vi "Check Error Core.vi"(8 "error in (no error)":errorcluster, 11 "Error Code":i32) -> (0 "error out":errorcluster)   [LabVIEW 2021, in "CIF_NI_CIPC.lvlib"]
doc: "This core VI is only called if an error exists. This is set for more effecient memory usage to not be reentrant."
uses:
  CIF_NI_CIPC.lvlib
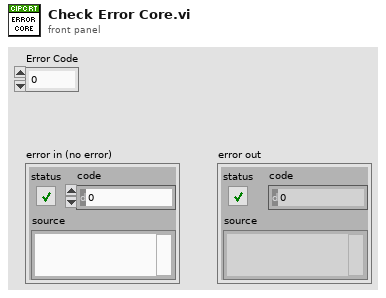
[diagram p1: front panel]
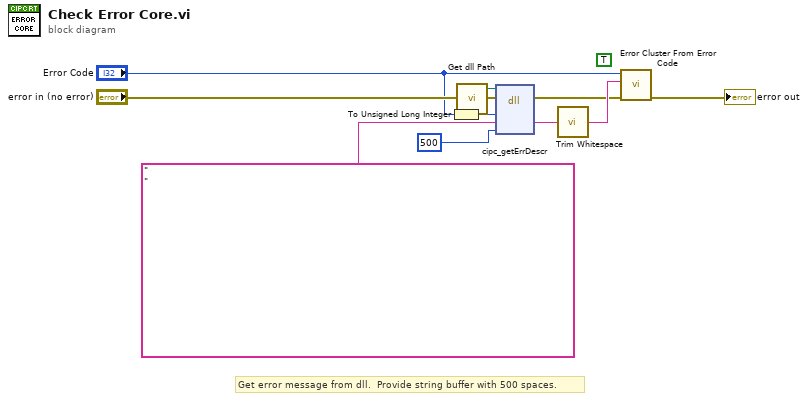
[diagram p0: block diagram]
diagram:
  (unwired) TRUE ("show call chain? (False)")
  # "Get error message from dll.  Provide string buffer with 500 spaces."
  n1 = To Unsigned Long Integer(number="Error Code") -> (unsigned 32bit integer=w8:u32)
  n2 = call "Get dll Path.vi"() -> ("appended path"=w10:path)  [unwired: 5 in]
  n3 = dll-call lib="libnicipc.*" fn="cipc_getErrDescr"(path in=w10, error in="error in (no error)", "err_code"=w8, "el_descr"="                                                                                                                                                                                                                                                                                                                                                                                                                                                                                                                    " ("string"), "el_descr_maxsize"=u32 500 ("dimension size")) -> (error out=w6:errorcluster, "el_descr"=w5:string)  [unwired: 4 in, 1 out]
  n4 = call <vilib>:"Trim Whitespace.vi"("string"=w5) -> ("trimmed string"=w9:string)  [unwired: 1 in]
  n5 = call <vilib>:"Error Cluster From Error Code.vi"("error in (no error)"=w6, "error message (\"\")"=w9, "error code (0)"="Error Code") -> ("error out"=→"error out":errorcluster)  [unwired: 6 in]
